vi "Close File.vi"(8 "error in (no error)":errorcluster, 11 "Spectrum Recorder in":refnum<class "Spectrum Recorder too.lvclass">) -> (0 "error out":errorcluster, 2 "Acquired Result.lvclass":refnum<class "Acquired Result.lvclass">, 3 "Spectrum Recorder out":refnum<class "Spectrum Recorder too.lvclass">)   [LabVIEW 2018, in "Spectrum Recorder too.lvclass"]
uses:
  Spectrum Recorder too.lvclass
  C:/github/LabActor/Worker/Worker.lvclass
  C:/github/LabActor/Template Module/Template Module.lvclass
  NHMFL_Core/Libraries/Instruments/Results/Acquired Result/Acquired Result.lvclass
  NHMFL_Core/Libraries/Instruments/Results/File Path Result/File Path Result.lvclass
  C:/github/NHMFL_Core/Libraries/Instruments/Results/Acquired Result/Acquired Result.lvclass
  Worker/Worker.lvclass/Worker.ctl
  Template Module/Template Module.lvclass/Template Module.ctl
  Spectrum Recorder too.lvclass/Spectrum Recorder too.ctl
  NHMFL_Core/Libraries/Instruments/Results/Acquired Result/Acquired Result.lvclass/Acquired Result.ctl
  Worker/Read Cycle count.vi
  Template Module/Read Logger.vi
  Worker/Write Cycle count.vi
  Template Module/Write Logger.vi
  NHMFL_Core/Libraries/Instruments/Results/Acquired Result/Write Cycle count.vi
  Loggers/Logger/Logger.lvclass
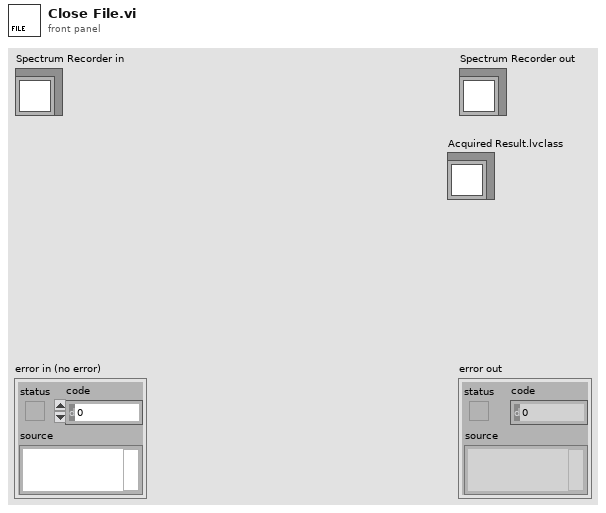
[diagram p1: front panel]
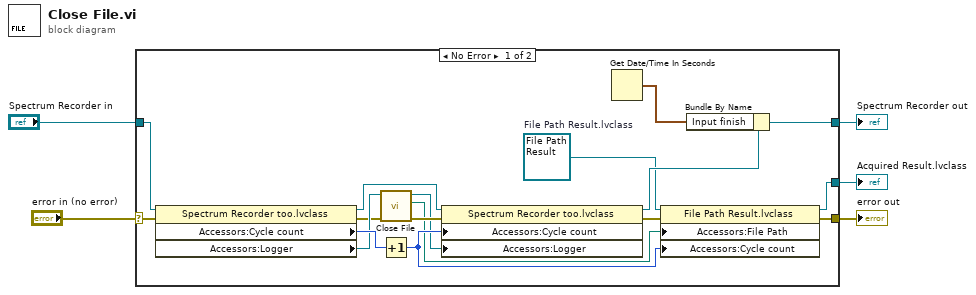
[diagram p0: block diagram]
diagram:
  n1 = case shown="No Error" "error in (no error)" {
    selector: "error in (no error)" -> [w21 w24]
    tunnel: [w18 w24] -> w4
    tunnel: [w19 w23] -> w2
    tunnel: "Spectrum Recorder in" -> [w22 w23]
    tunnel: [w20 _] -> w1
    frame No Error {
      w13 = refnum<class "File Path Result.lvclass"> refnum  # File Path Result.lvclass
      n2 = property class="Spectrum Recorder too.lvclass"(reference=w22, error in=w21) -> (reference out=w17:refnum<class "Spectrum Recorder too.lvclass">, error out=w9:errorcluster, "Accessors:Cycle count"=w16:i32, "Accessors:Logger"=w10:refnum<class "Logger.lvclass">)
      n3 = call-dynamic "Close File.vi"("error in (no error)"=w9, "Logger in"=w10) -> ("error out"=w8:errorcluster, "File Path"=w6:path, "Logger out"=w7:refnum<class "Logger.lvclass">)  [unwired: 6 in, 1 out]
      n4 = Increment(x=w16) -> (x+1=w11:i32)
      n5 = property class="Spectrum Recorder too.lvclass"(reference=w17, error in=w8, "Accessors:Cycle count"=w11, "Accessors:Logger"=w7) -> (reference out=w14:refnum<class "Spectrum Recorder too.lvclass">, error out=w15:errorcluster)
      n6 = Get Date/Time In Seconds() -> (seconds since 1Jan1904=w12:timestamp)
      n7 = property class="File Path Result.lvclass"(reference=w13, error in=w15, "Accessors:File Path"=w6, "Accessors:Cycle count"=w11) -> (reference out=w20:refnum<class "File Path Result.lvclass">, error out=w18:errorcluster)
      n8 = Bundle By Name(cluster=w14, "Input finish"=w12) -> (w19:refnum<class "Spectrum Recorder too.lvclass">)
    }
    frame Error {
    }
  }
  "error out" <- w4
  "Spectrum Recorder out" <- w2
  "Acquired Result.lvclass" <- w1
